vi "Get Macros Setup.vi"(8 "error in (no error)":errorcluster, 11 "Motions Configuration in":refnum<class "Motions Configuration.lvclass">) -> (0 "error out":errorcluster, 1 "Macros List":cluster{"enabled?":bool, "macro name":string}[](array[cluster]), 2 "Macro LUT (Name->Macro)":variant, 3 "Motions Configuration out":refnum<class "Motions Configuration.lvclass">)   [LabVIEW 2016, in "Hardware.lvlib" / "Motions.lvlib" / "Motions Configuration.lvclass"]
uses:
  <userlib>/Common Components/Hardware/Abstract System/Motions/Motions Config/Motions Configuration.lvclass
  <userlib>/Common Components/Hardware/Abstract System/Motions/Motions Config/Motions Configuration.lvclass/Motions Configuration.ctl
  <userlib>/Common Components/Hardware/Abstract System/Motions/Motions/Motions.lvclass/Motions.ctl
  <userlib>/Common Components/Hardware/Abstract System/Motions/Motions/Motions.lvclass
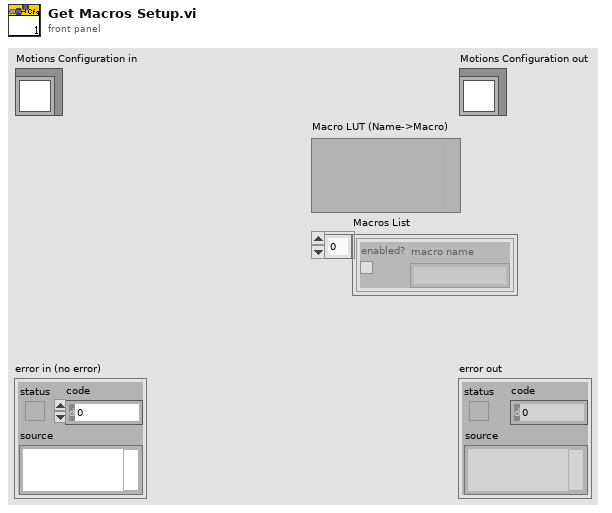
[diagram p1: front panel]
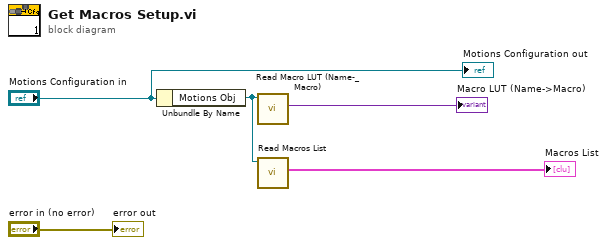
[diagram p0: block diagram]
diagram:
  n1 = Unbundle By Name("Motions Configuration in") -> ("Motions Obj"=w3:refnum<class "Motions.lvclass">)
  n2 = call <userlib>:"Read Macro LUT (Name-_Macro).vi"("Motions in"=w3) -> ("Macro LUT (Name->Macro)"=→"Macro LUT (Name->Macro)":variant)  [unwired: 9 in, 1 out]
  n3 = call <userlib>:"Read Macros List.vi"("Motions in"=w3) -> ("Macros List"=→"Macros List":cluster{"enabled?":bool, "macro name":string}[])  [unwired: 9 in, 1 out]
  "error out" <- "error in (no error)"
  "Motions Configuration out" <- "Motions Configuration in"
